vi "[R]_ZYX.vi"(2 "Marker 2":dbl[](array[numeric]), 3 "Origin":dbl[](array[numeric]), 4 "Marker 1":dbl[](array[numeric])) -> (0 "[R]T":dbl[][](array[numeric]), 1 "[R]":dbl[][](array[numeric]))   [LabVIEW 2010]
uses:
  <vilib>/Analysis/baseanly.llb/Unit Vector (DBL).vi
  <vilib>/Analysis/NI_AALBase.lvlib
  <vilib>/Analysis/NI_AALPro.lvlib
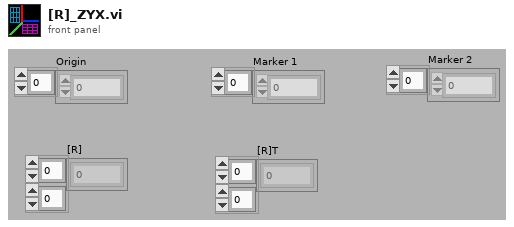
[diagram p1: front panel]
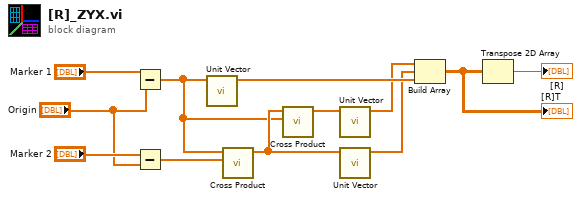
[diagram p0: block diagram]
diagram:
  n1 = Subtract(x="Marker 1", y="Origin") -> (x-y=w1:dbl[])
  n2 = Subtract(x="Marker 2", y="Origin") -> (x-y=w3:dbl[])
  n3 = call-poly <vilib>:"Unit Vector.vi"("Input Vector"=w1) -> ("Unit Vector"=w9:dbl[])  [unwired: 8 in, 2 out]
  n4 = call <vilib>:"Cross Product.vi"("B Vector"=w3, "A Vector"=w1) -> ("Cross Product"=w2:dbl[])  [unwired: 8 in, 1 out]
  n5 = call <vilib>:"Cross Product.vi"("B Vector"=w1, "A Vector"=w2) -> ("Cross Product"=w10:dbl[])  [unwired: 8 in, 1 out]
  n6 = call-poly <vilib>:"Unit Vector.vi"("Input Vector"=w10) -> ("Unit Vector"=w7:dbl[])  [unwired: 8 in, 2 out]
  n7 = call-poly <vilib>:"Unit Vector.vi"("Input Vector"=w2) -> ("Unit Vector"=w8:dbl[])  [unwired: 8 in, 2 out]
  n8 = Build Array(w7, w8, w9) -> (w12:dbl[][])
  "[R]T" <- w12
  n9 = Transpose 2D Array(2D array=w12) -> (transposed array=→"[R]":dbl[][])
